vi "Error Strings Global Internal.vi"() -> ()   [LabVIEW 2025]
panel:
  out "7051":string="<b>Invalid Data Types</b>\n\nInvalid measurement configurations:\n%s\n\nInvalid measurement results:\n%s\n\nThe data type of these controls or indicators are not supported by the Measurement Service. For arrays, enums, and rings, the underlying representation must be a supported data type.\n\nSee \"https://www.ni.com/r/measurementlinkdatatypes\" for details."
  out "7050":string="<b>Invalid Data Types</b>\n\nInvalid measurement configurations:\n%s\n\nInvalid measurement results:\n%s\n\nThe data type of these controls or indicators are not supported by the Measurement Service. For arrays, enums, and rings, the underlying representation must be a supported data type.\n\nSee \"https://www.ni.com/r/measurementlinkdatatypes\" for details."
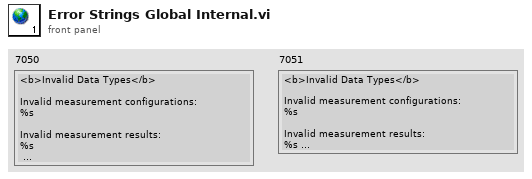
[diagram p1: front panel]
diagram:
